vi "Inject Attribute List.vi"(6 "Attributes Ref":refnum<data-value>, 8 "error in (no error)":errorcluster, 11 "Start Low Pressure Wax in":refnum<class "Start Low Pressure Wax.lvclass">) -> (0 "error out":errorcluster, 3 "Start Low Pressure Wax out":refnum<class "Start Low Pressure Wax.lvclass">)   [LabVIEW 2019, in "Start Low Pressure Wax.lvclass"]
uses:
  <vilib>/gpm_packages/@cs/Car-wash/Source/Process Steps/Start Low Pressure Wax/Start Low Pressure Wax.lvclass
  <vilib>/gpm_packages/@cs/lookup-table/Source/LookupTable/LookupTable.lvclass
  <vilib>/gpm_packages/@cs/lookup-table/Source/LookupTable/LookupTable.lvclass/LookupTable.ctl
  <vilib>/gpm_packages/@cs/Car-wash/Source/Process Steps/Start Low Pressure Wax/Start Low Pressure Wax.lvclass/Start Low Pressure Wax.ctl
  ece17c9a-c4ad-4727-8e8b-9859ae002eb0.vi
  <vilib>/gpm_packages/@cs/lookup-table/Source/LookupTable/Read Table Reference.vi
  ece17c9a-c4ad-4727-8e8b-9859ae002eb0.vi/a585ebf6-862c-427e-978c-b67117c33868.vi
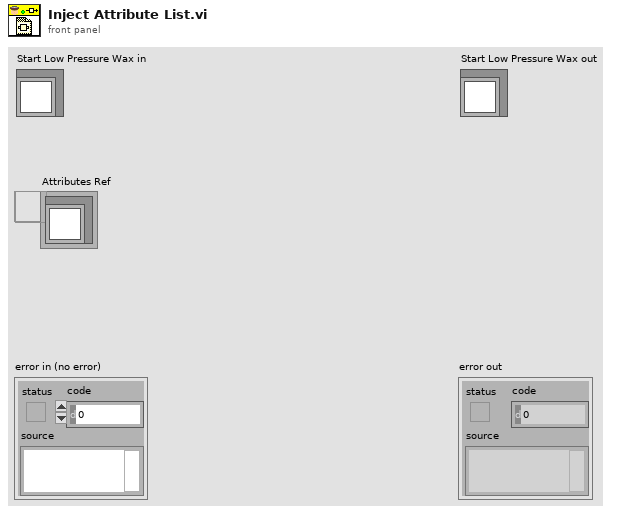
[diagram p1: front panel]
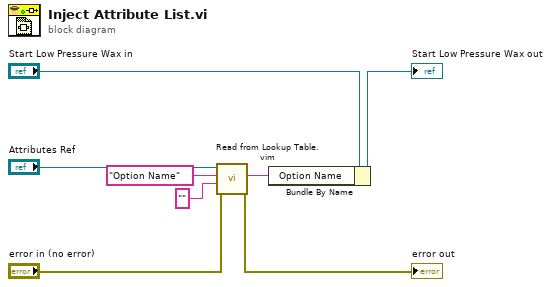
[diagram p0: block diagram]
diagram:
  n1 = call "Read from Lookup Table.vim"("error in (no error)"="error in (no error)", "Type"="", "Item Name"="Option Name", "LookupTable Reference"="Attributes Ref") -> ("error out"=→"error out":errorcluster, "Value"=w6:string)  [unwired: 4 in, 2 out]
  n2 = Bundle By Name(cluster="Start Low Pressure Wax in", "Option Name"=w6) -> (→"Start Low Pressure Wax out":refnum<class "Start Low Pressure Wax.lvclass">)
